vi "SetTriggering.vi"(0 "instrument handle out":refnum<k15>, 1 "trigger slope":T1 caption="trigger slope (Positive)", 2 "Triggering?":bool, 5 "Trigger Level":dbl, 9 "trigger source":T2="0" caption="trigger source (Channel 0)", 11 "error in":errorcluster, 12 "Analog Triggering":bool, 13 "Triggering:Trigger Modifier":i32(ring)=2 items=["None"=1, "Auto Trigger"=2]) -> (4 "instrument handle out 2":refnum<k15>, 15 "error out":errorcluster)   [LabVIEW 2012]
uses:
  <instrlib>/niScope/Controls/niScope trigger source.ctl
  <instrlib>/niScope/Controls/niScope trigger slope.ctl
  <instrlib>/niScope/Controls/niScope trigger coupling.ctl
  <instrlib>/niScope/Configure/Trigger/niScope Configure Trigger Immediate.vi
  <instrlib>/niScope/Configure/Trigger/niScope Configure Trigger Edge.vi
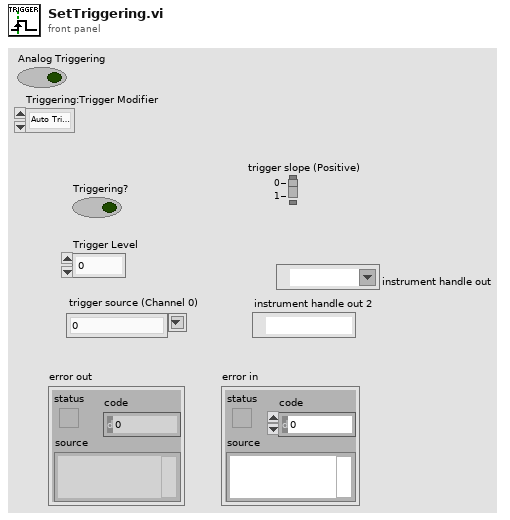
[diagram p1: front panel]
types:
  T1 = typedef "niScope trigger slope.ctl" = i32
  T2 = typedef "niScope trigger source.ctl" = string
  T3 = typedef "niScope trigger coupling.ctl" = u16
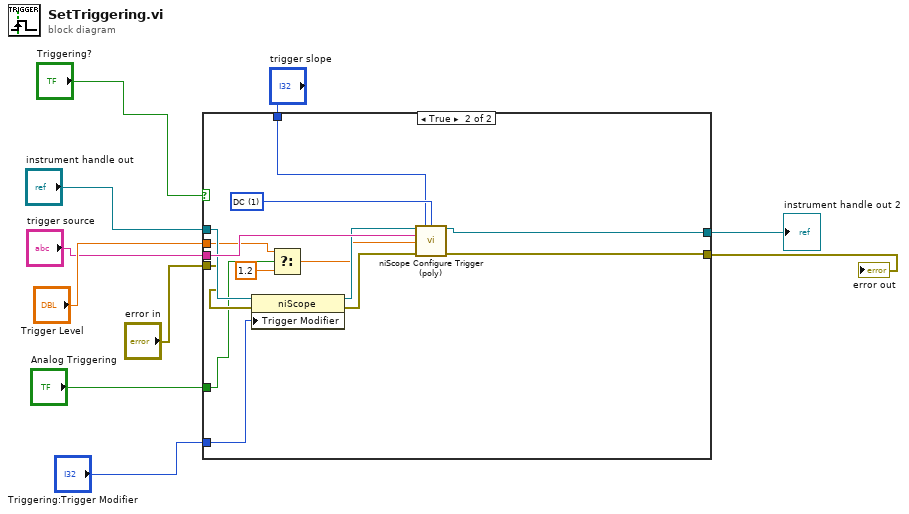
[diagram p0: block diagram]
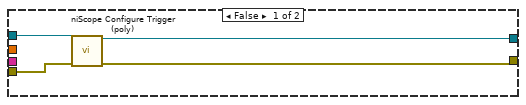
[diagram p2: hidden frame]
diagram:
  n1 = case shown="True" "Triggering?" {
    tunnel: [w13 w21] -> w4
    tunnel: [w14 w20] -> w5
    tunnel: "instrument handle out" -> [w12 w25]
    tunnel: "Trigger Level" -> [_ w18]
    tunnel: "trigger source" -> [_ w28]
    tunnel: "error in" -> [w11 w24]
    tunnel: "trigger slope" -> [_ w26]
    tunnel: "Analog Triggering" -> [_ w16]
    tunnel: "Triggering:Trigger Modifier" -> [_ w15]
    frame False {
      n2 = call-poly <instrlib>:"niScope Configure Trigger (poly).vi"("instrument handle"=w12, "error in"=w11) -> ("instrument handle out"=w13:refnum<k15>, "error out"=w14:errorcluster)  [unwired: 12 in]
    }
    frame True {
      w27 = T3 1 items=["AC"=0, "DC"=1, "HF Reject"=3, "LF Reject"=4, "AC Plus HF Reject"=1001] ("trigger coupling")
      n3 = property class="niScope"(reference=w25, error in=w24, "Trigger Modifier"=w15) -> (reference out=w23:refnum<k15>, error out=w22:errorcluster)
      n4 = Select(t=w18, s=w16, f=1.2) -> (s? t:f=w19:dbl)
      n5 = call-poly <instrlib>:"niScope Configure Trigger (poly).vi"("instrument handle"=w23, "trigger slope"=w26, "trigger coupling"=w27, "trigger source"=w28, "trigger level"=w19, "error in"=w22) -> ("instrument handle out"=w21:refnum<k15>, "error out"=w20:errorcluster)  [unwired: 8 in]
    }
  }
  "error out" <- w5
  "instrument handle out 2" <- w4
